vi "Faults.GetChannelFaultValue.vi"(10 "Channel Name":string, 11 "GatewayIP":string) -> (0 "error out":errorcluster, 2 "Faulted":bool, 3 "Fault Value":dbl)   [LabVIEW 2013, in "MiscHelperVIs.lvlib"]
uses:
  MiscHelperVIs.lvlib
  <vilib>/NI Veristand/Execution/ChannelFaultManager/NI_VS ChannelFault ExecutionAPI.lvlib
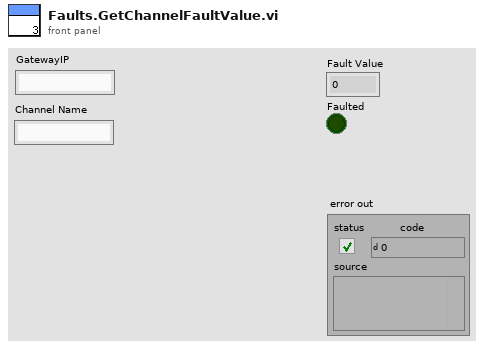
[diagram p1: front panel]
types:
  T1 = typedef "NI_VS ChannelFault ExecutionAPI.lvlib/ChannelFaultAPI.ctl" = refnum<k24>
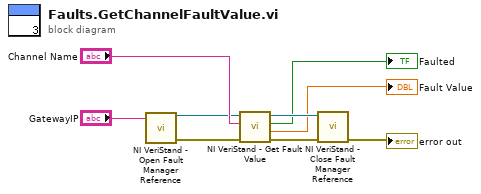
[diagram p0: block diagram]
diagram:
  n1 = call <vilib>:"NI VeriStand - Open Fault Manager Reference.vi"("Gateway IP Address (\"\": localhost)"="GatewayIP") -> ("error out"=w8:errorcluster, "ChannelFault"=w6:T1)  [unwired: 9 in]
  n2 = call <vilib>:"NI VeriStand - Get Fault Value.vi"("error in (no error)"=w8, "Channel"="Channel Name", "ChannelFault in"=w6) -> ("error out"=w5:errorcluster, "Fault Value"=→"Fault Value":dbl, "Faulted"=→"Faulted":bool, "ChannelFault out"=w4:T1)  [unwired: 5 in]
  n3 = call <vilib>:"NI VeriStand - Close Fault Manager Reference.vi"("error in (no error)"=w5, "ChannelFault"=w4) -> ("error out"=→"error out":errorcluster)  [unwired: 9 in]
